vi "FFT.vi"() -> ()   [LabVIEW 2016]
uses:
  controls/Enum.ctl
  <vilib>/Analysis/2dsp.llb/Power Spectrum (DBL).vi
  <vilib>/Utility/error.llb/Error Cluster From Error Code.vi
  <vilib>/rvi/errors/niLvFpgaAdjustHostInterfaceError.vi
  <vilib>/rvi/interface/nirviReadWriteControl/nirviReadWriteControl.xnode
  controls/FPGAVIreferenceTypeDef.ctl
  FPGA Bitfiles/qnmController797_usbRIO_controllerFPGAUS_vDhBWyMsd7A.lvbitx
  NiFpgaLv.dll
  <vilib>/Analysis/NI_AALPro.lvlib
  <vilib>/Analysis/NI_AALBase.lvlib
panel:
  out "abs(x)":dbl[](graph)
  out "1/x":dbl
  out "Waveform Graph 3":cluster{i32, "sample length":i32, dbl[]}(graph)
  out "Waveform Graph":cluster{i32, dbl, "Power Spectrum":dbl[]}(graph)
  in  "sample length":i32=1000
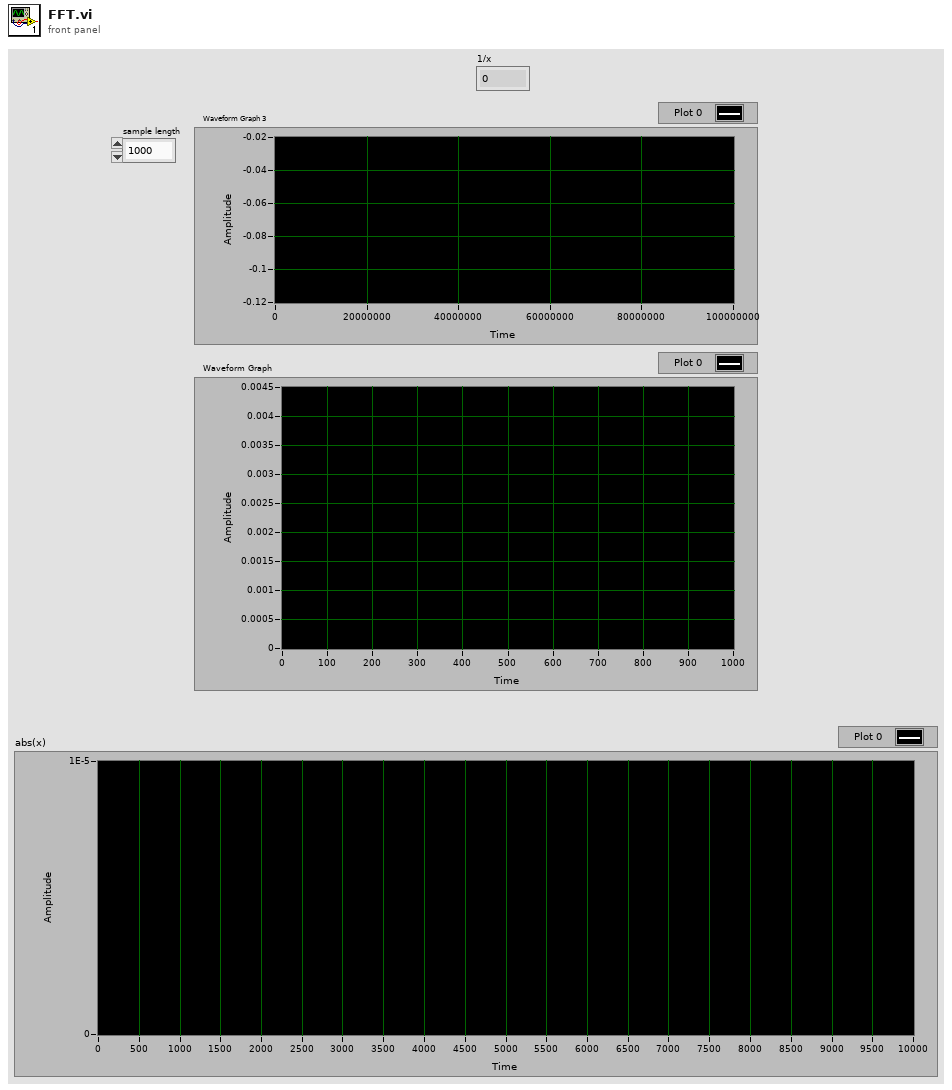
[diagram p1: front panel]
types:
  T1 = typedef "Enum.ctl" = enum16{"Init", "Read", "Write"}
  T2 = typedef "FPGAVIreferenceTypeDef.ctl" = refnum<k20>
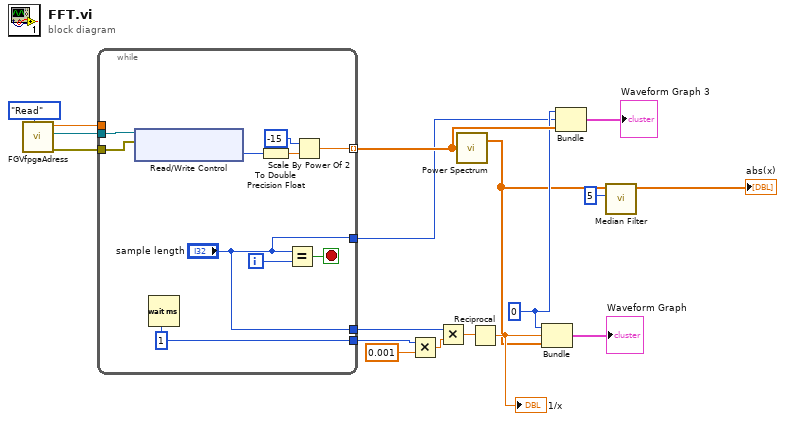
[diagram p0: block diagram]
diagram:
  w8 = 0
  n1 = call "FGVfpgaAdress.vi"("Enum"=Enum."Read") -> ("error out"=w16:errorcluster, "FPGA VI Reference Out"=w17:T2, "voltageRange(+/-)Out"=w15:dbl)  [unwired: 6 in, 2 out]
  n2 = while {
    tunnel: w17 -> [w28]
    tunnel: w16 -> [w27]
    tunnel: w15 -> [_]
    tunnel: [w21] -> w9 mode=indexing
    tunnel: ["sample length"] -> w4
    tunnel: [w20] -> w7
    tunnel: ["sample length"] -> w14
    i -> [w24]
    stop <- w23 stop-if-true
    w20 = u32 1 ("milliseconds to wait")
    n3 = xnode "Read/Write Control"("FPGA VI Reference In"=w28, "error in"=w27) -> ("aio.s.slowVertical"=w22:i16)  [unwired: 2 out]
    n4 = Wait (ms)(milliseconds to wait=w20) -> ()  [unwired: 1 out]
    n5 = To Double Precision Float(number=w22) -> (double precision float=w26:dbl)
    n6 = Equal?(x="sample length", y=w24) -> (x = y?=w23:bool)
    n7 = Scale By Power Of 2(n=i16 -15, x=w26) -> (x*2^n=w21:dbl)
  }
  n8 = Multiply(x=w7, y=0.001) -> (x*y=w6:dbl)
  n9 = Multiply(x=w14, y=w6) -> (x*y=w13:dbl)
  n10 = call-poly <vilib>:"Power Spectrum.vi"("X"=w9) -> ("Power Spectrum"=w1:dbl[])  [unwired: 1 out]
  n11 = Reciprocal(x=w13) -> (1/x=w12:dbl)
  "1/x" <- w12
  n12 = Bundle(w8, w12, "Power Spectrum"=w1) -> (→"Waveform Graph":cluster{i32, dbl, "Power Spectrum":dbl[]})  [unwired: 1 in]
  n13 = Bundle(w8, "sample length"=w4, w9) -> (→"Waveform Graph 3":cluster{i32, "sample length":i32, dbl[]})  [unwired: 1 in]
  n14 = call <vilib>:"Median Filter.vi"("left rank"=5, "X"=w1) -> ("Filtered X"=→"abs(x)":dbl[])  [unwired: 8 in, 1 out]
